vi "Pipeline Change.vi"(7 "Description":string, 8 "Command Info In":T2, 11 "Pipeline":T1) -> (0 "Command Info Out":T2)   [LabVIEW 2018]
doc: "This template is useful for immediate subsystem actions that do not need deadband filtering\n\nBe sure to right-click and select New from Template and save with a new command name."
uses:
  <vilib>/Rock Robotics/WPI/Framework/Command Status Info.ctl
  <vilib>/Rock Robotics/WPI/Framework/Completion Status.ctl
  <vilib>/Rock Robotics/WPI/Framework/Completion Notifier.ctl
  Pipeline Index.ctl
  Implementation/Limelight Setpoints.ctl
  Implementation/Limelight Operations.ctl
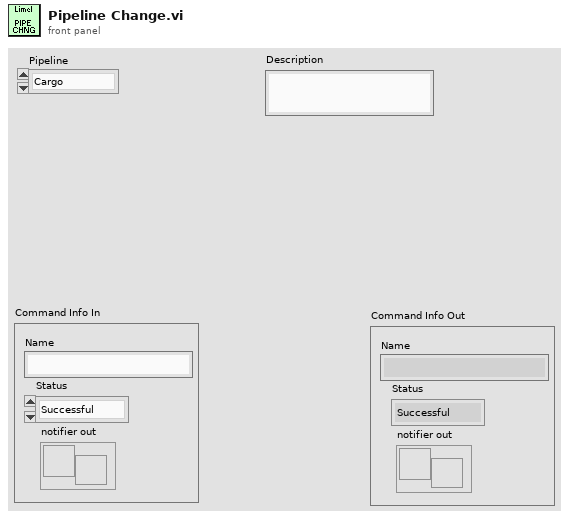
[diagram p1: front panel]
types:
  T1 = typedef "Pipeline Index.ctl" = enum16{"Cargo", "Hatch", "Vision"}
  T2 = typedef "Command Status Info.ctl" = cluster{"Name":string, "Status":T3, "notifier out":T4}
  T3 = typedef "Completion Status.ctl" = enum16{"Successful", "Aborted", "Incomplete"}
  T4 = typedef "Completion Notifier.ctl" = refnum<notifier>
  T5 = typedef "Limelight Setpoints.ctl" = cluster{"Operation":T6, "Setpoint":dbl, "Duration":dbl}
  T6 = typedef "Limelight Operations.ctl" = enum16{"Reserve", "Read Current", "Immediate", "Pipeline Change"}
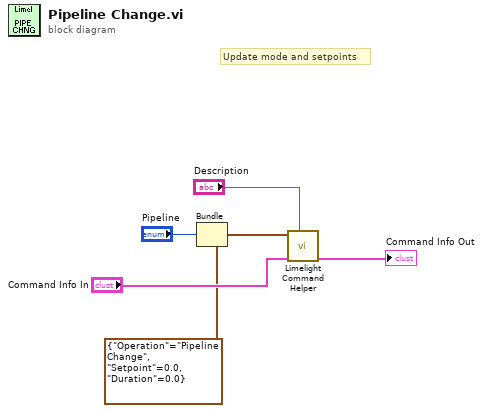
[diagram p0: block diagram]
diagram:
  # "Update mode and setpoints"
  n1 = Bundle(cluster=T5 {"Operation"=enum."Pipeline Change", "Setpoint"=0.0, "Duration"=0.0} ("SubSystem Data"), "Setpoint"="Pipeline") -> (w2:T5)  [unwired: 2 in]
  n2 = call "Limelight Command Helper.vi"("Description"="Description", "Command Info In"="Command Info In", "SubSystem Data"=w2) -> ("Command Info Out"=→"Command Info Out":T2)  [unwired: 6 in, 2 out]
